vi "losslessCompression.vi"(5 "Image":T1, 7 "error in (no error)":errorcluster) -> (0 "Data String":string, 3 "error out":errorcluster)   [LabVIEW 2011]
uses:
  IMAQ Image.ctl
panel:
  out "length":i32
  out "number of replacements":i32
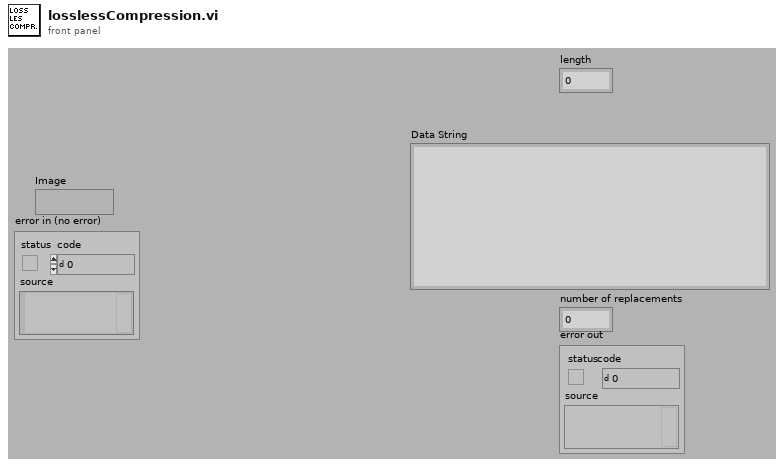
[diagram p1: front panel]
types:
  T1 = typedef "IMAQ Image.ctl" = refnum<image>
  T2 = typedef "Image Type" = u32
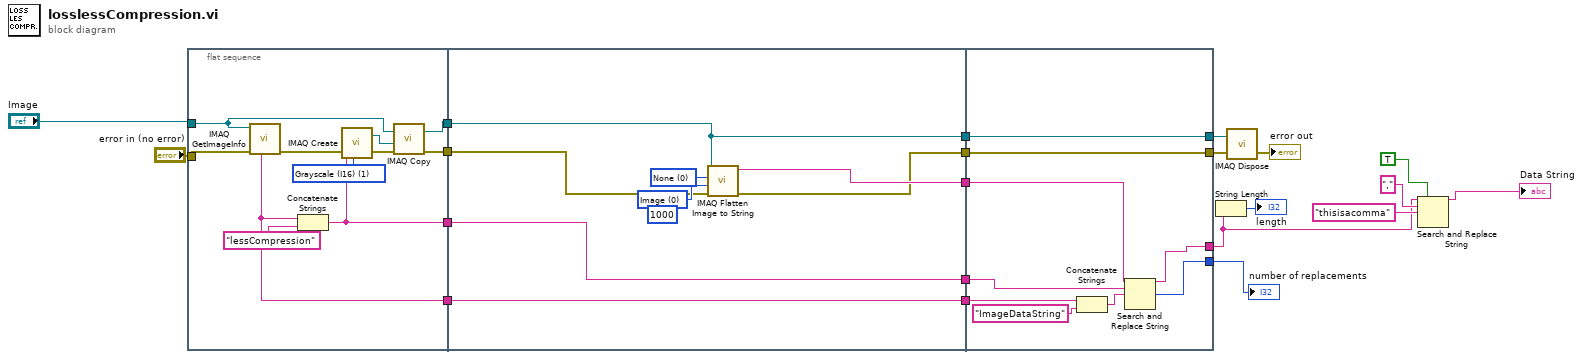
[diagram p0: block diagram]
diagram:
  n1 = flat-sequence {
    tunnel: "error in (no error)" -> [w28]
    tunnel: "Image" -> [w30]
    tunnel: [w29] -> w14
    tunnel: [w25] -> w10
    tunnel: [w24] -> w8
    tunnel: [w23] -> w7
    tunnel: w14 -> [w38]
    tunnel: [w35] -> w13
    tunnel: [w38] -> w12
    tunnel: [w37] -> w11
    tunnel: w10 -> [w36]
    tunnel: [w34] -> w9
    tunnel: w8 -> [w34]
    tunnel: w7 -> [w33]
    tunnel: [w33] -> w6
    tunnel: [w48] -> w16
    tunnel: [w49] -> w18
    tunnel: [w44] -> w21
    tunnel: [w43] -> w2
    tunnel: w13 -> [w49]
    tunnel: w12 -> [w48]
    tunnel: w11 -> [w42]
    tunnel: w9 -> [w46]
    tunnel: w6 -> [w45]
    frame #0 {
      w32 = T2 1 items=["Grayscale (U8)", "Grayscale (I16)", "Grayscale (SGL)", "Complex (CSG)", "RGB (U32)", "HSL (U32)", "RGB (U64)", "Grayscale (U16)"] ("Image Type")
      n2 = call "IMAQ GetImageInfo"("error in (no error)"=w28, "Image"=w30) -> ("error out"=w27:errorcluster, "Image Name"=w23:string)  [unwired: 2 in, 6 out]
      n3 = Concatenate Strings(w23, "lessCompression" ("string")) -> (w24:string)
      n4 = call "IMAQ Create"("Image Name"=w24, "Image Type"=w32, "error in (no error)"=w27) -> ("New Image"=w31:T1, "error out"=w26:errorcluster)  [unwired: 2 in]
      n5 = call "IMAQ Copy"("error in (no error)"=w26, "Image Dst"=w31, "Image Src"=w30) -> ("error out"=w25:errorcluster, "Image Dst Out"=w29:T1)  [unwired: 3 in]
    }
    frame #1 {
      w39 = 0 items=["Image", "Image and Vision Info", "Reference to Image"] ("Type of Flatten (Image and Vision Info)")
      (unwired) 1000 ("Quality (750)")
      w40 = 0 items=["None", "JPEG", "PACKED BINARY"] ("Compression (None)")
      n6 = call "IMAQ Flatten Image to String"("error in (no error)"=w36, "Type of Flatten (Image and Vision Info)"=w39, "Compression (None)"=w40, "Image"=w38) -> ("error out"=w35:errorcluster, "Data String"=w37:string)  [unwired: 6 in]
    }
    frame #2 {
      n7 = Concatenate Strings(w45, "ImageDataString" ("replace string (\"\")")) -> (w47:string)
      n8 = Search and Replace String(input string=w42, search string=w46, replace string=w47) -> (result string=w43:string, number of replacements=w44:i32)  [unwired: 5 in, 2 out]
    }
  }
  n9 = String Length(string=w2) -> (length=→"length":i32)
  n10 = call "IMAQ Dispose"("Image"=w16, "error in (no error)"=w18) -> ("error out"=→"error out":errorcluster)  [unwired: 4 in]
  n11 = Search and Replace String(replace all?=TRUE ("replace all? (F)"), input string=w2, search string=",", replace string="thisisacomma" ("replace string (\"\")")) -> (result string=→"Data String":string)  [unwired: 4 in, 3 out]
  "number of replacements" <- w21
